vi "Correct_Mistakes_101-Reconstruct_Tracks-1.vi"(4 "error IN":errorcluster, 5 "[IN] Clusters for Re\nconstructed Tracks":T1, 7 "[IN] Number of Subtracks":i32) -> (0 "error OUT":errorcluster, 1 "[OUT] Clusters for Re\nconstructed Tracks":T1)   [LabVIEW 2013]
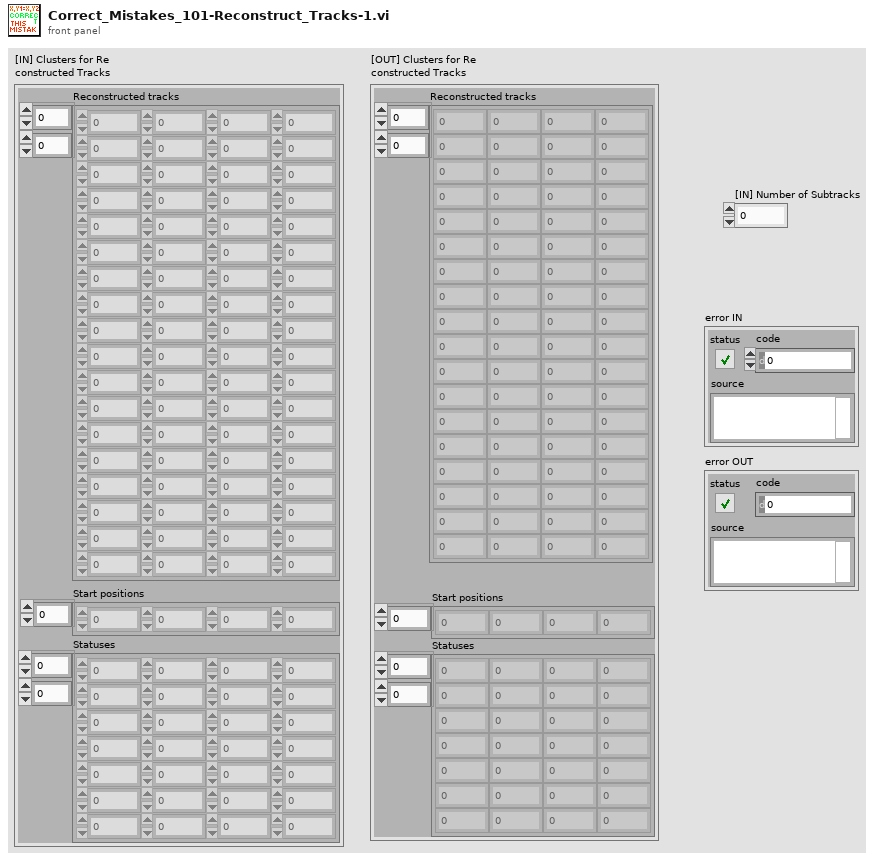
[diagram p1: front panel]
types:
  T1 = cluster{"Reconstructed tracks":dbl[][], "Start positions":i32[], "Statuses":i16[][]}
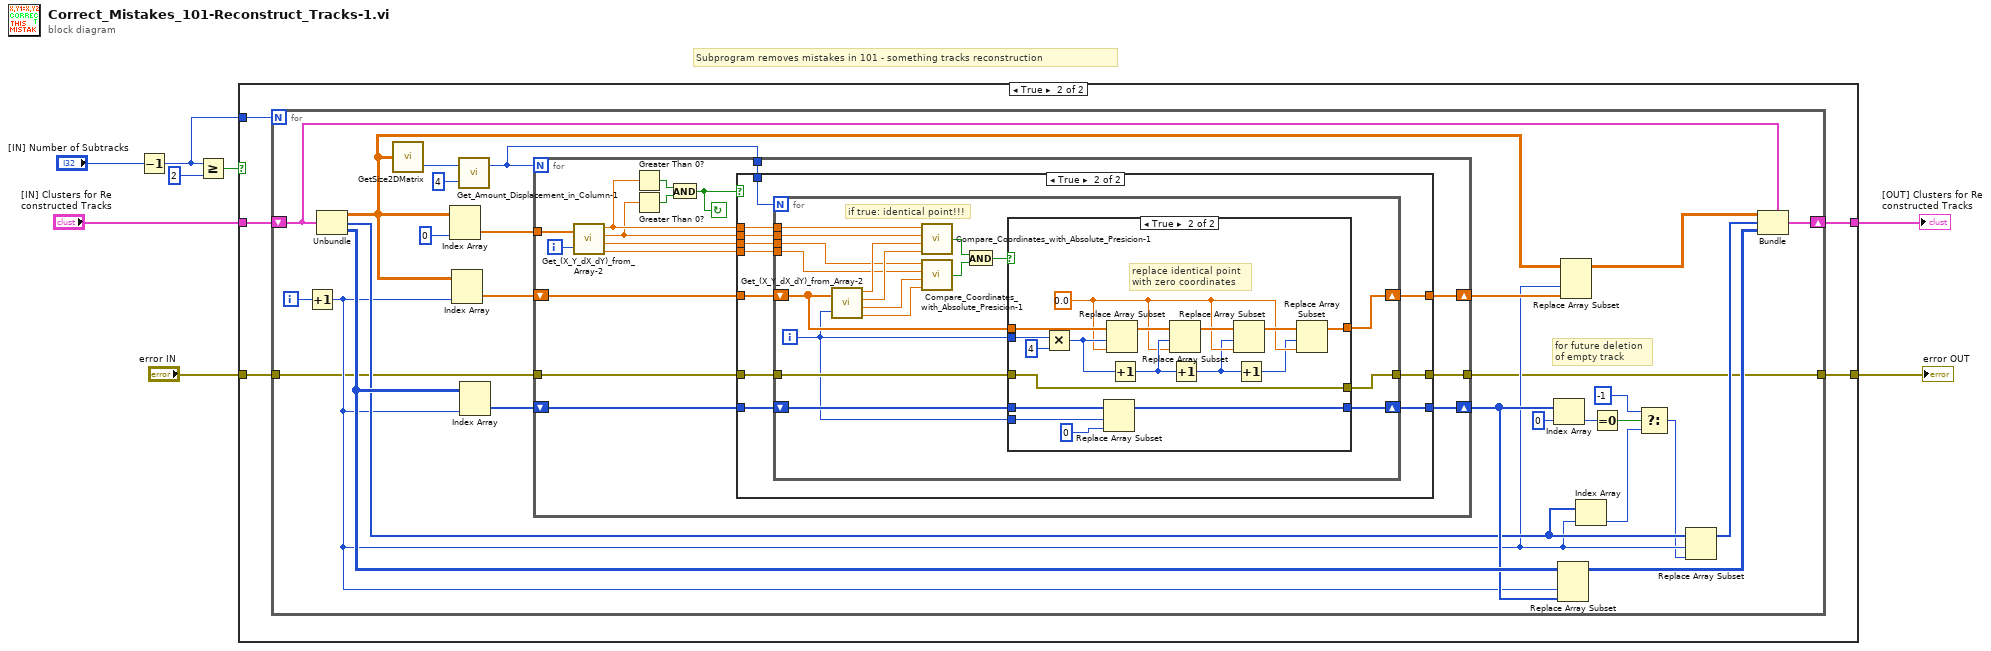
[diagram p0: block diagram]
diagram:
  # "Subprogram removes mistakes in 101 - something tracks reconstruction"
  n1 = Decrement(x="[IN] Number of Subtracks") -> (x-1=w4:i32)
  n2 = Greater Or Equal?(x=w4, y=2) -> (x >= y?=w5:bool)
  n3 = case shown="True" w5 {
    tunnel: "[IN] Clusters for Re\nconstructed Tracks" -> [w10 w15]
    tunnel: w4 -> [_ w14]
    tunnel: [w10 w13] -> w3
    tunnel: "error IN" -> [w9 w12]
    tunnel: [w9 w11] -> w1
    frame False {
    }
    frame True {
      n4 = for {
        N: w14 -> [_]
        shift-right: [w19] -> w13
        shift-left: w15 -> [w24]
        tunnel: w12 -> [w18]
        tunnel: [w17] -> w11
        i -> [w42]
        # "for future deletion\nof empty track"
        n5 = Increment(x=w42) -> (x+1=w26:i32)
        n6 = Unbundle(w24) -> ("Reconstructed tracks"=w35:dbl[][], "Start positions"=w27:i32[], "Statuses"=w32:i16[][])
        n7 = call "GetSize2DMatrix.vi"("Array IN (2D)"=w35) -> ("# Rows"=w39:i32)  [unwired: 1 out]
        n8 = Index Array(array=w35, index (col)=0) -> (element=w38:dbl[])  [unwired: 1 in]
        n9 = Index Array(array=w35, index (col)=w26) -> (element=w37:dbl[])  [unwired: 1 in]
        n10 = call "Get_Amount_Displacement_in_Column-1.vi"("multiplier"=4 ("y"), "# Rows"=w39) -> ("Displ amount"=w16:i32)  [unwired: 1 out]
        n11 = Index Array(array=w32, index (col)=w26) -> (element=w36:i16[])  [unwired: 1 in]
        n12 = for {
          N: w16 -> [_]
          tunnel: w38 -> [w52]
          shift-right: [w55] -> w34
          shift-left: w37 -> [w58]
          shift-right: [w56] -> w31
          shift-left: w36 -> [w57]
          tunnel: w18 -> [w54]
          tunnel: [w53] -> w17
          tunnel: w16 -> [w43]
          i -> [w51]
          stop <- w44 continue-if-true
          n13 = call "Get_(X_Y_dX_dY)_from_Array-2.vi"("(X,Y,dX,dY)"=w52, "Index of Displacement"=w51) -> ("X"=w50:dbl, "Y"=w49:dbl, "dX"=w46:dbl, "dY"=w45:dbl)
          n14 = Greater Than 0?(x=w50) -> (x > 0?=w48:bool)
          n15 = Greater Than 0?(x=w49) -> (x > 0?=w47:bool)
          n16 = And(x=w48, y=w47) -> (x .and. y?=w44:bool)
          n17 = case shown="True" w44 {
            tunnel: w58 -> [w60 w71]
            tunnel: w57 -> [w59 w65]
            tunnel: [w59 w62] -> w56
            tunnel: [w60 w63] -> w55
            tunnel: w54 -> [w61 w66]
            tunnel: [w61 w64] -> w53
            tunnel: w50 -> [_ w70]
            tunnel: w49 -> [_ w69]
            tunnel: w46 -> [_ w68]
            tunnel: w45 -> [_ w67]
            tunnel: w43 -> [_ w72]
            frame False {
            }
            frame True {
              n18 = for {
                N: w72 -> [_]
                tunnel: w70 -> [w88]
                tunnel: w69 -> [w87]
                tunnel: w68 -> [w84]
                tunnel: w67 -> [w83]
                shift-right: [w76] -> w63
                shift-left: w71 -> [w79]
                tunnel: w66 -> [w78]
                tunnel: [w74] -> w64
                shift-right: [w73] -> w62
                shift-left: w65 -> [w77]
                i -> [w75]
                # "if true: identical point!!!"
                n19 = call "Get_(X_Y_dX_dY)_from_Array-2.vi"("(X,Y,dX,dY)"=w79, "Index of Displacement"=w75) -> ("X"=w85:dbl, "Y"=w86:dbl, "dX"=w82:dbl, "dY"=w81:dbl)
                n20 = call "Compare_Coordinates_with_Absolute_Presicion-1.vi"("X 1"=w88, "Y 1"=w87, "X 2"=w85, "Y 2"=w86) -> ("[OUT] Same coordinates?"=w89:bool)  [unwired: 1 in]
                n21 = call "Compare_Coordinates_with_Absolute_Presicion-1.vi"("X 1"=w84, "Y 1"=w83, "X 2"=w82, "Y 2"=w81) -> ("[OUT] Same coordinates?"=w90:bool)  [unwired: 1 in]
                n22 = And(x=w89, y=w90) -> (x .and. y?=w80:bool)
                n23 = case shown="True" w80 {
                  tunnel: w79 -> [w93 w110]
                  tunnel: w75 -> [_ w108]
                  tunnel: w77 -> [w92 w106]
                  tunnel: [w92 w101] -> w73
                  tunnel: [w93 w96] -> w76
                  tunnel: w78 -> [w91 w95]
                  tunnel: [w91 w95] -> w74
                  tunnel: w75 -> [_ w94]
                  frame False {
                  }
                  frame True {
                    w99 = 0.0 ("new element/subarray")
                    # "replace identical point \nwith zero coordinates"
                    n24 = Multiply(x=w108, y=4) -> (x*y=w105:i32)
                    n25 = Replace Array Subset(array=w106, new element=i16 0 ("new element/subarray"), index=w94) -> (w101:i16[])
                    n26 = Replace Array Subset(array=w110, new element=w99, index=w105) -> (w107:dbl[])
                    n27 = Increment(x=w105) -> (x+1=w102:i32)
                    n28 = Replace Array Subset(array=w107, new element=w99, index=w102) -> (w103:dbl[])
                    n29 = Increment(x=w102) -> (x+1=w98:i32)
                    n30 = Replace Array Subset(array=w103, new element=w99, index=w98) -> (w100:dbl[])
                    n31 = Increment(x=w98) -> (x+1=w97:i32)
                    n32 = Replace Array Subset(array=w100, new element=w99, index=w97) -> (w96:dbl[])
                  }
                }
              }
            }
          }
        }
        n33 = Index Array(array=w31, index=0) -> (element=w28:i16)
        n34 = Replace Array Subset(array=w32, new element=w31, index (col)=w26) -> (w20:i16[][])  [unwired: 1 in]
        n35 = Replace Array Subset(array=w35, new element=w34, index (col)=w26) -> (w23:dbl[][])  [unwired: 1 in]
        n36 = Index Array(array=w27, index=w26) -> (element=w25:i32)
        n37 = Equal To 0?(x=w28) -> (x = 0?=w30:bool)
        n38 = Select(t=-1 ("new element/subarray"), s=w30, f=w25) -> (s? t:f=w22:i32)
        n39 = Replace Array Subset(array=w27, new element=w22, index=w26) -> (w21:i32[])
        n40 = Bundle(cluster=w24, "Reconstructed tracks"=w23, "Start positions"=w21, "Statuses"=w20) -> (w19:T1)
      }
    }
  }
  "[OUT] Clusters for Re\nconstructed Tracks" <- w3
  "error OUT" <- w1
